vi "Example.vi"() -> ()   [LabVIEW 2019]
uses:
  Test Bench Tools.lvlib
panel:
  in  "Stop":bool
  in  "Launch Test":bool
  out "SerialNumber":string
  out "Test Result":bool
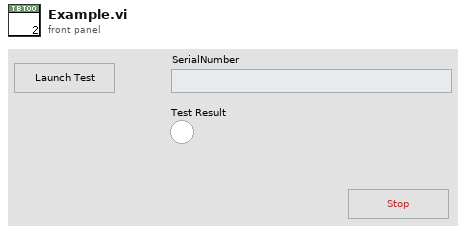
[diagram p1: front panel]
types:
  T1 = enum16{"Station 1", "Station 2", "Station 3", "Station 4"}
  T2 = cluster{"new reference":refnum<k24>, "Array":refnum<k27>[], "Mgessage":refnum<user-event>}
  T3 = enum32{"Invalid", "Standard", "Closed", "Hidden", "Minimized", "Maximized"}
  T4 = enum32{"invalid app kind", "Development System", "Run Time System", "Student Edition", "Embedded LabVIEW", "Evaluation", "Custom"}
  T5 = cluster{"Core":cluster{"Current VI Reference":refnum<vi>, "Close Panel on Exit?":bool}, "Your Boolean data":bool, "Your string data":string, "hWnd":u32}
  T6 = cluster{"Current VI Reference":refnum<vi>, "Close Panel on Exit?":bool}
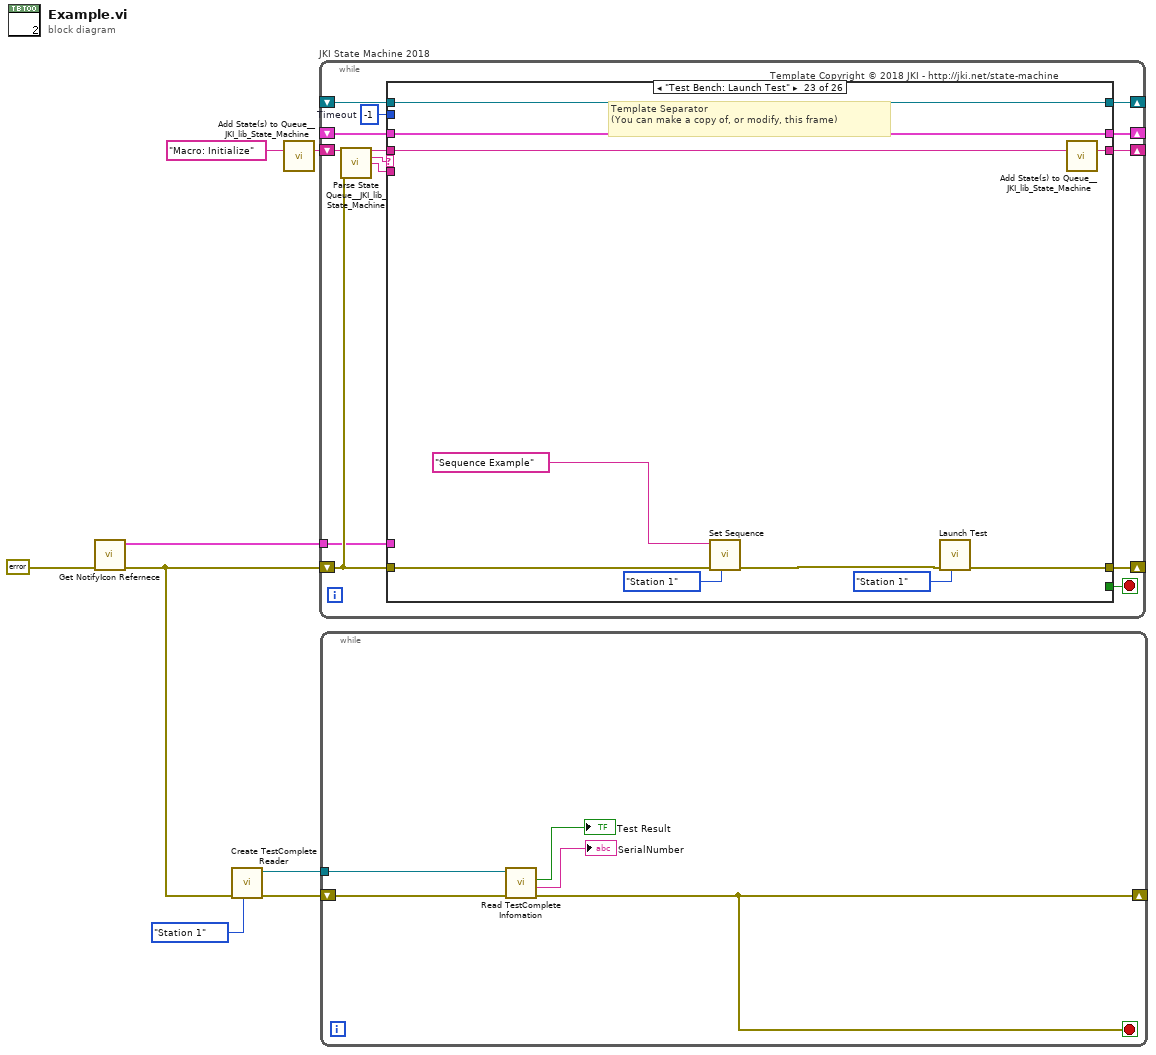
[diagram p0: block diagram]
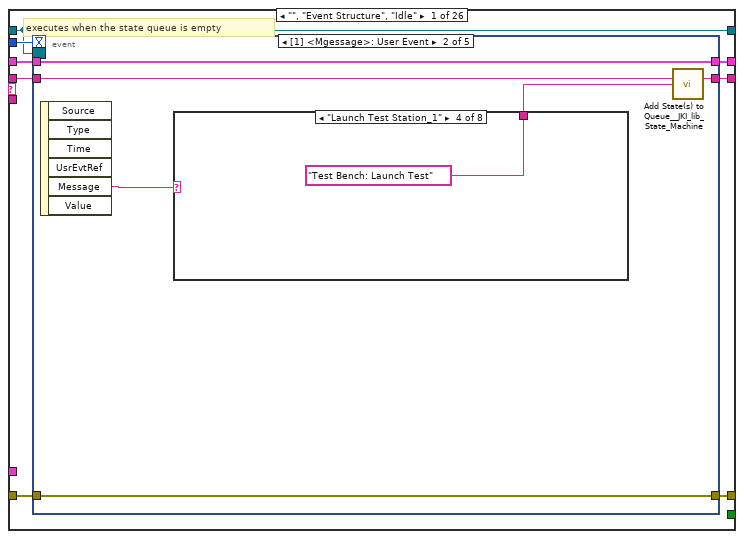
[diagram p2: hidden frame]
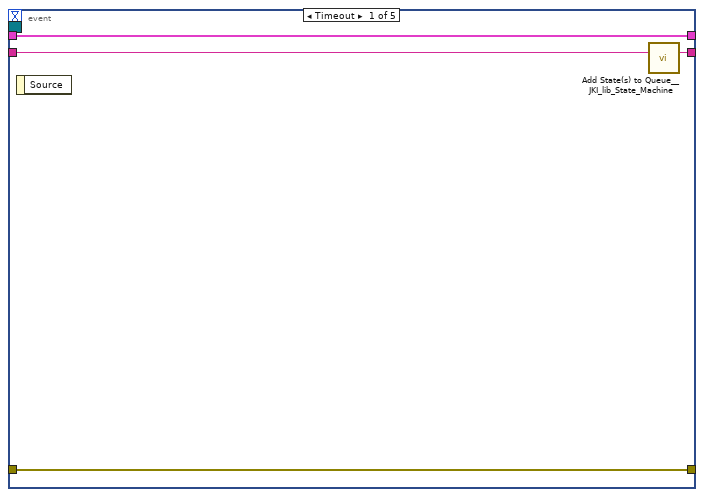
[diagram p3: hidden frame]
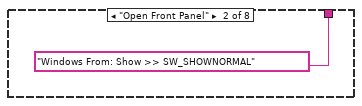
[diagram p5: hidden frame]
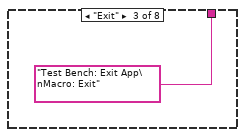
[diagram p6: hidden frame]
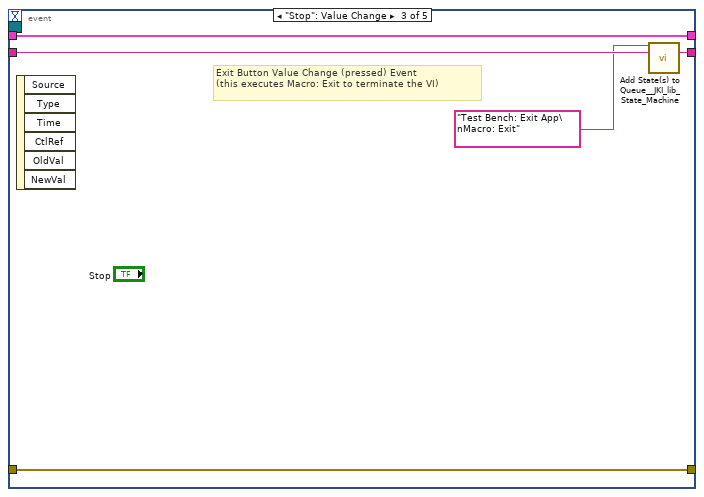
[diagram p11: hidden frame]
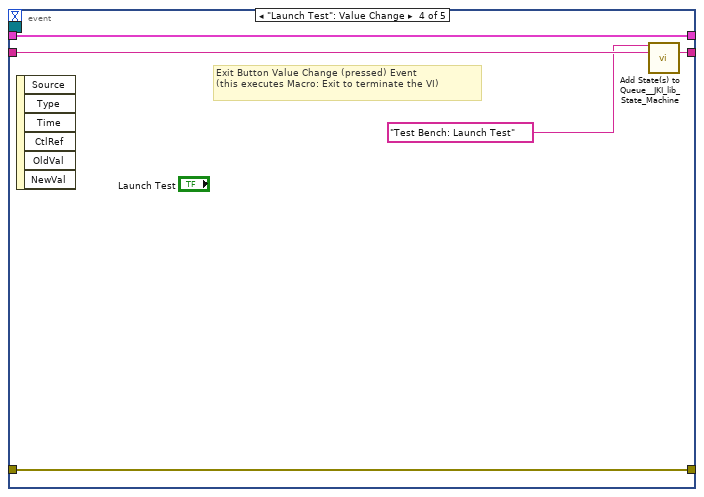
[diagram p12: hidden frame]
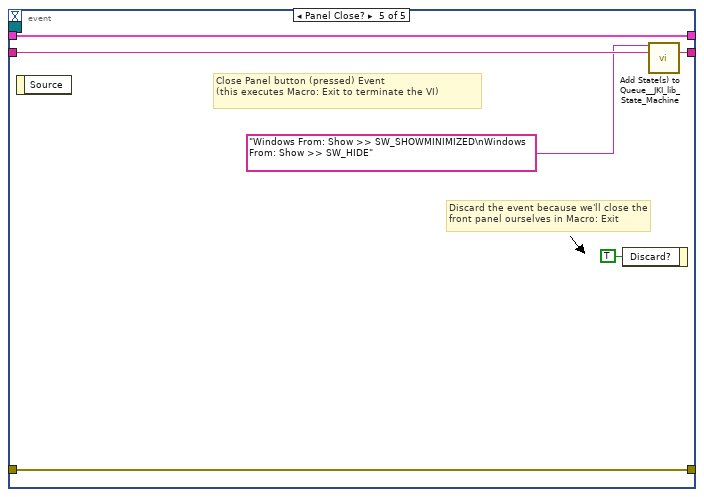
[diagram p13: hidden frame]
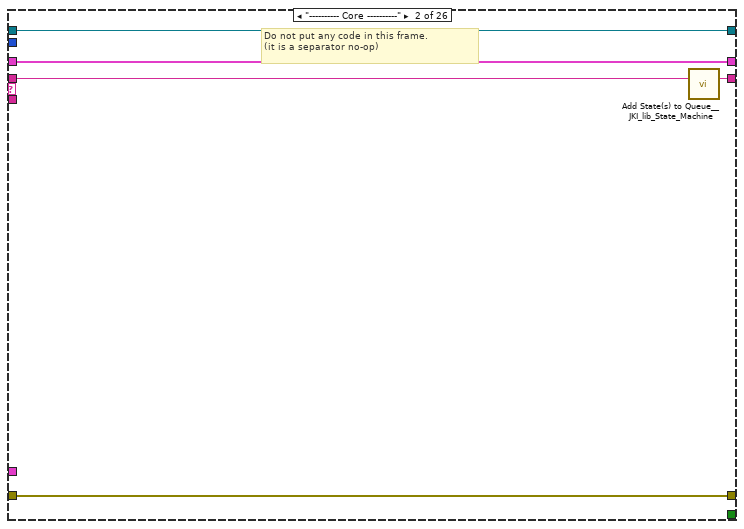
[diagram p14: hidden frame]
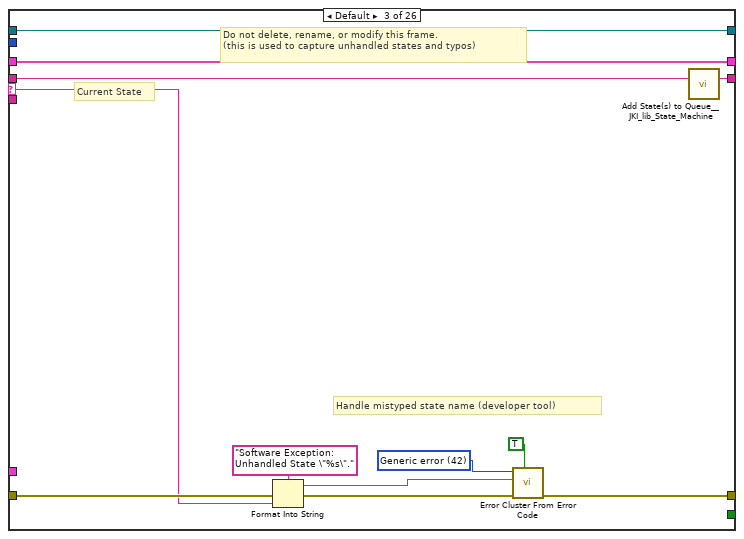
[diagram p15: hidden frame]
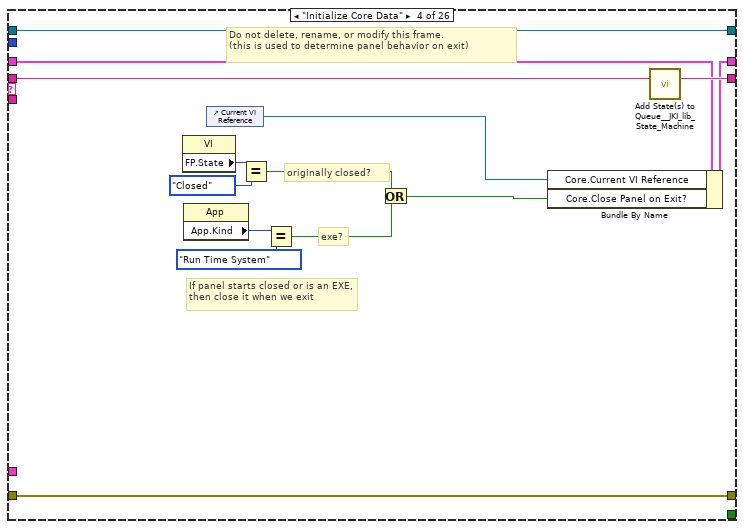
[diagram p16: hidden frame]
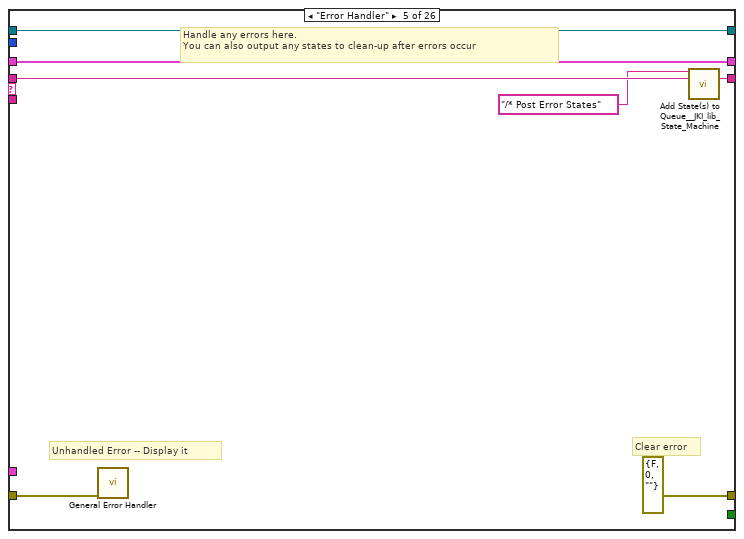
[diagram p17: hidden frame]
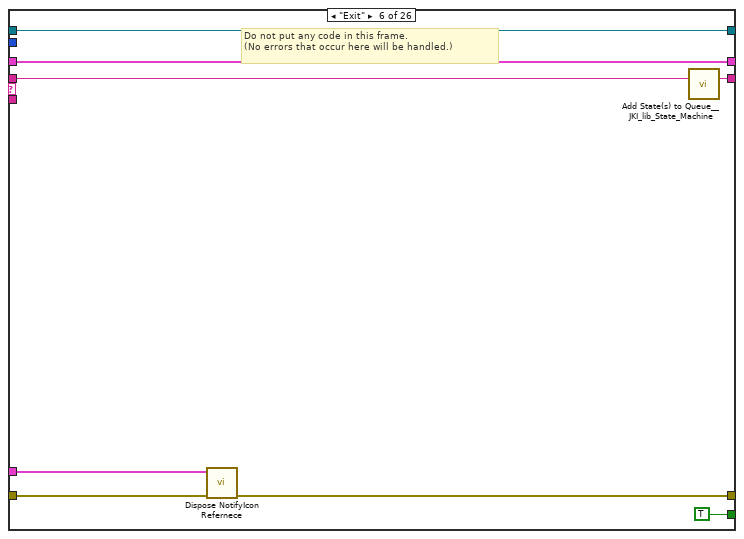
[diagram p18: hidden frame]
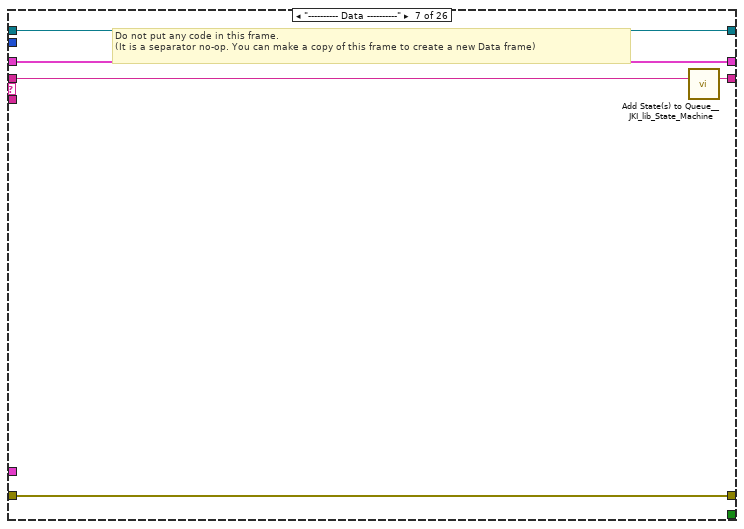
[diagram p19: hidden frame]
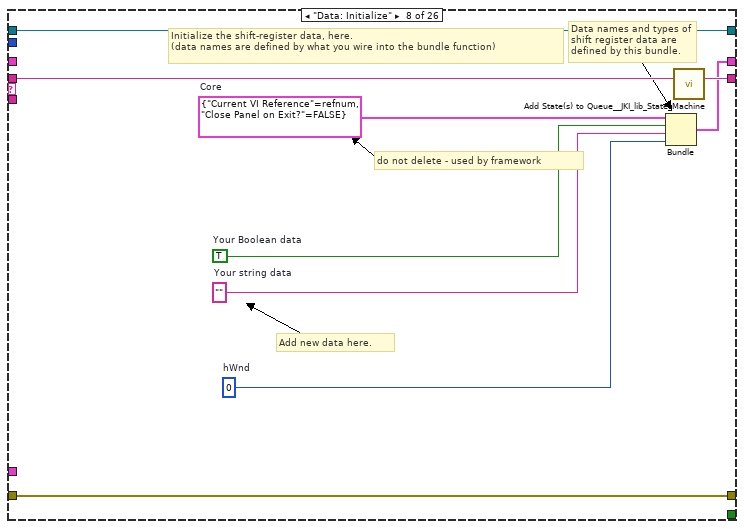
[diagram p20: hidden frame]
diagram:
  n1 = call "Get NotifyIcon Refernece.vi"("error in (no error)"=errorcluster {"status"=FALSE, "code"=0, "source"=""} ("error out")) -> ("error out"=w2:errorcluster, "reference out"=w1:T2)  [unwired: 9 in]
  n2 = call "Create TestComplete Reader.vi"("Station"=T1."Station 1", "error in (no error)"=w2) -> ("error out"=w6:errorcluster, "reader endpoint"=w4:refnum<k21>)  [unwired: 8 in]
  n3 = call <vilib>:"Add State(s) to Queue__JKI_lib_State_Machine.vi"("State(s) in (\"\")"="Macro: Initialize") -> ("States Out"=w8:string)  [unwired: 14 in]
  n4 = while "JKI State Machine 2018" {
    shift-right: [w15] -> _
    shift-left: _ -> [w14]
    shift-right: [w18] -> _
    shift-left: w2 -> [w12]
    shift-right: [w17] -> _
    shift-left: w8 -> [w19]
    shift-right: [w11] -> _
    shift-left: _ -> [w10]
    tunnel: w1 -> [w9]
    stop <- w16 stop-if-true
    w13 = -1  # Timeout
    # "Template Copyright © 2018 JKI - http://jki.net/state-machine"
    n5 = call <vilib>:"Parse State Queue__JKI_lib_State_Machine.vi"("State Queue"=w19, "Error In (no error)"=w12) -> ("Remaining States"=w21:string, "Current State"=w22:string, "Arguments"=w20:string)  [unwired: 11 in]
    n6 = case shown="\"Test Bench: Launch Test\"" w22 {
      selector: w22 -> [_ _ w66 _ _ _ _ _ _ _ _ _ _ _ _ _ _ _ _ _ _ _ _ _ _ _]
      tunnel: w21 -> [w30 w64 w70 w90 w97 w105 w110 w119 w126 w131 w139 w145 w150 w155 w162 w174 w244 w250 w261 w266 w274 w281 w291 w296 w304 w313]
      tunnel: w20 -> [_ _ _ _ _ _ _ _ _ _ _ _ _ _ w157 w168 _ _ _ _ _ _ _ _ w297 _]
      tunnel: w14 -> [w28 w61 w68 w83 w94 w103 w107 _ w121 w128 w137 w143 w147 w153 w160 w170 w241 w247 w258 w263 w272 w279 w289 w293 w299 w307]
      tunnel: [w27 w62 w72 w87 errorcluster {"status"=FALSE, "code"=0, "source"=""} ("error out") w98 w108 w116 w122 w129 w135 w140 w148 w152 w158 w171 w242 w248 w259 w264 w270 w277 w288 w292 w300 w309] -> w18
      tunnel: w12 -> [w26 w62 w71 w87 w93 w99 w108 w116 w123 w129 w134 w141 w148 w152 w159 w172 w242 w248 w259 w264 w271 w278 w285 w292 w301 w310]
      tunnel: [w29 w63 w69 w89 w96 w104 w109 w118 w125 w130 w138 w144 w149 w154 w161 w173 w243 w249 w260 w265 w273 w280 w290 w295 w303 w312] -> w17
      tunnel: [_ _ _ _ _ TRUE _ _ _ _ _ _ _ _ _ _ _ _ _ _ _ _ _ _ _ _] -> w16
      tunnel: [w25 w61 w68 w88 w94 w103 w107 w117 w121 w128 w137 w143 w147 w153 w160 w170 w241 w247 w258 w263 w272 w279 w289 w293 w299 w305] -> w15
      tunnel: w13 -> [w24 _ _ _ _ _ _ _ _ _ _ _ _ _ _ _ _ _ _ _ _ _ _ _ _ _]
      tunnel: [w23 w60 w65 w77 w91 w101 w106 w112 w120 w127 w136 w142 w146 w151 w156 w167 w240 w245 w251 w262 w268 w275 w286 w294 w302 w311] -> w11
      tunnel: w10 -> [w23 w60 w65 w77 w91 w101 w106 w112 w120 w127 _ w142 w146 w151 w156 w167 w240 w245 w251 w262 w268 w275 w286 w294 w302 w311]
      tunnel: w9 -> [_ _ _ _ _ w100 _ _ _ _ w133 _ _ _ _ _ _ _ _ _ _ _ _ _ _ _]
      frame "", "Event Structure", "Idle" {
        # "executes when the state queue is empty"
        n7 = event shown="[1] <Mgessage>: User Event" {
          selector: w23 -> [_ _ _ _ _]
          dyn-events: _ -> [_ _ _ _ _]
          timeout: w24 -> [_ _ _ _ _]
          tunnel: w30 -> [w34 w40 w48 w53 w59]
          tunnel: [w33 w39 w47 w52 w58] -> w29
          tunnel: w28 -> [w31 w37 w45 w50 w56]
          tunnel: [w32 w38 w46 w51 w57] -> w27
          tunnel: w26 -> [w32 w38 w46 w51 w57]
          tunnel: [w31 w37 w45 w50 w56] -> w25
          event Timeout {
            n8 = event-data() -> ()  [unwired: 1 in, 1 out]
            n9 = call <vilib>:"Add State(s) to Queue__JKI_lib_State_Machine.vi"("State(s) in (\"\")"=w34) -> ("States Out"=w33:string)  [unwired: 14 in]
          }
          event User Event {
            n10 = event-data() -> ("Message"=w36:string)  [unwired: 1 in, 5 out]
            n11 = case shown="\"Launch Test Station_1\"" w36 {
              tunnel: [_ "Windows From: Show >> SW_SHOWNORMAL" "Test Bench: Exit App\nMacro: Exit" "Test Bench: Launch Test" _ _ _ _] -> w35
              frame "Idle", Default {
              }
              frame "Open Front Panel" {
              }
              frame "Exit" {
              }
              frame "Launch Test Station_1" {
              }
              frame "Launch Test Station_2" {
              }
              frame "Launch Test Station_3" {
              }
              frame "Launch Test Station_4" {
              }
              frame "Change Product Model" {
              }
            }
            n12 = call <vilib>:"Add State(s) to Queue__JKI_lib_State_Machine.vi"("State(s) in (\"\")"=w40, "State(s) at Back (\"\")"=w35) -> ("States Out"=w39:string)  [unwired: 13 in]
          }
          event "Stop": Value Change {
            # "Exit Button Value Change (pressed) Event\n(this executes Macro: Exit to terminate the VI)"
            n13 = event-data() -> ()  [unwired: 1 in, 6 out]
            n14 = call <vilib>:"Add State(s) to Queue__JKI_lib_State_Machine.vi"("State(s) in Front (\"\")"="Test Bench: Exit App\nMacro: Exit", "State(s) in (\"\")"=w48) -> ("States Out"=w47:string)  [unwired: 13 in]
          }
          event "Launch Test": Value Change {
            # "Exit Button Value Change (pressed) Event\n(this executes Macro: Exit to terminate the VI)"
            n15 = event-data() -> ()  [unwired: 1 in, 6 out]
            n16 = call <vilib>:"Add State(s) to Queue__JKI_lib_State_Machine.vi"("State(s) in Front (\"\")"="Test Bench: Launch Test", "State(s) in (\"\")"=w53) -> ("States Out"=w52:string)  [unwired: 13 in]
          }
          event Panel Close? {
            # "Discard the event because we'll close the front panel ourselves in Macro: Exit"
            # "Close Panel button (pressed) Event\n(this executes Macro: Exit to terminate the VI)"
            n17 = event-data() -> ()  [unwired: 1 in, 1 out]
            n18 = event-data("Discard?"=TRUE) -> ()  [unwired: 1 in, 1 out]
            n19 = call <vilib>:"Add State(s) to Queue__JKI_lib_State_Machine.vi"("State(s) in Front (\"\")"="Windows From: Show >> SW_SHOWMINIMIZED\nWindows From: Show >> SW_HIDE", "State(s) in (\"\")"=w59) -> ("States Out"=w58:string)  [unwired: 13 in]
          }
        }
      }
      frame "---------- Core ----------" {
        # "Do not put any code in this frame.\n(it is a separator no-op)"
        n20 = call <vilib>:"Add State(s) to Queue__JKI_lib_State_Machine.vi"("State(s) in (\"\")"=w64) -> ("States Out"=w63:string)  [unwired: 14 in]
      }
      frame Default {
        w75 = 42 items=["No error", "Argument error", "Memory is full", "Out of zone", "End of file", "File already open", "Generic file I/O error", "File not found", "File permission error", "Disk is full", "Duplicate path", "Too many files open", "System feature not enabled", "Resource file not found", "Cannot add resource", "Resource not found", "Image not found", "Image memory error", "Pen does not exist", "Config type invalid", "Config token not found", "Config parse error", "Config memory error", "Bad external code format", "Bad external code offset", "External code not present", "Null window", "Destroy window error", "Null menu", "Print aborted", "Bad print record", "Print driver error", "Windows error during printing", "Memory error during printing", "Print dialog error", "Generic print error", "Invalid device refnum", "Device not found", "Device parameter error", "Device unit error", "Cannot open device", "Device call aborted", "Generic error", "Cancelled by user", "Object ID too low", "Object ID too high", "Object not in heap", "Unknown heap", "Unknown object (invalid DefProc)", "Unknown object (DefProc not in table)", "Message out of range", "Invalid (null) method", "Unknown message", "Manager call not supported", "Bad address", "Network operation in progress", "Network operation timed out", "Connection is busy", "Network attribute not supported", "Network error", "Address in use", "System out of memory", "Connection aborted", "Connection refused", "Not connected", "Already connected", "Connection closed", "Initialization error (interapplication manager)", "Bad occurrence", "Wait on unbound occurrence handler", "Occurrence queue overflow", "Datalog type conflict", "Unused", "Unrecognized type (interapplication manager)", "Memory corrupt", "Failed to make temporary DLL", "Old CIN version", "Drag socket not found", "Failed to load drop-object", "Failed to register OLE object", "Failed to release OLE object", "Format specifier type mismatch", "Unknown format specifier", "Too few format specifiers", "Too many format specifiers", "Scan failed", "Newer CIN version", "Error converting to variant", "Runtime menu error", "Password tampered", "Variant attribute not found", "Incompatible variant data type", "Event data is not available", "Event Store is not present", "Occurrence is not found", "Event Queue is not created", "Event info is not available", "Refnum passed is NULL", "Error retrieving Class GUID", "Error retrieving CoClass GUID", "Error retrieving TypeLib GUID.", "Bad built application magic bytes.", "Specific driver is different from the specific driver associated with the Logical Name.", "There is no session opened to the class driver.", "Max Error", "MAX - Error with config objects", "MAX - Error loading configuration", "MAX - Group not supported"]
        # "Current State"
        # "Do not delete, rename, or modify this frame.\n(this is used to capture unhandled states and typos)"
        # "Handle mistyped state name (developer tool)"
        n21 = Format Into String(format string="Software Exception: Unhandled State \"%s\"." ("message"), error in=w71, w66) -> (resulting string=w74:string, error out=w73:errorcluster)  [unwired: 1 in]
        n22 = call <vilib>:"Error Cluster From Error Code.vi"("show call chain? (False)"=TRUE, "error in (no error)"=w73, "error message (\"\")"=w74, "error code (0)"=w75) -> ("error out"=w72:errorcluster)  [unwired: 5 in]
        n23 = call <vilib>:"Add State(s) to Queue__JKI_lib_State_Machine.vi"("State(s) in (\"\")"=w70) -> ("States Out"=w69:string)  [unwired: 14 in]
      }
      frame "Initialize Core Data" {
        # "Do not delete, rename, or modify this frame.\n(this is used to determine panel behavior on exit)"
        # "originally closed?"
        # "exe?"
        # "If panel starts closed or is an EXE, then close it when we exit"
        n24 = property class="VI"() -> ("FP.State"=w80:T3)  [unwired: 2 in, 2 out]
        n25 = property class="App"() -> ("App.Kind"=w86:T4)  [unwired: 2 in, 2 out]
        n26 = control-ref of="Current VI Reference"() -> (w81:refnum<vi>)
        n27 = Equal?(x=w80, y=T3."Closed" ("Front Panel Window:State")) -> (x = y?=w78:bool)
        n28 = Equal?(x=w86, y=T4."Run Time System" ("Application:Kind")) -> (x = y?=w84:bool)
        n29 = Or(x=w78, y=w84) -> (x .or. y?=w82:bool)
        n30 = Bundle By Name(cluster=w83, "Core.Current VI Reference"=w81, "Core.Close Panel on Exit?"=w82) -> (w88:T5)
        n31 = call <vilib>:"Add State(s) to Queue__JKI_lib_State_Machine.vi"("State(s) in (\"\")"=w90) -> ("States Out"=w89:string)  [unwired: 14 in]
      }
      frame "Error Handler" {
        # "Unhandled Error -- Display it"
        # "Handle any errors here.\nYou can also output any states to clean-up after errors occur"
        # "Clear error"
        n32 = call <vilib>:"General Error Handler.vi"("error in (no error)"=w93) -> ()  [unwired: 10 in, 5 out]
        n33 = call <vilib>:"Add State(s) to Queue__JKI_lib_State_Machine.vi"("State(s) in Front (\"\")"="/* Post Error States", "State(s) in (\"\")"=w97) -> ("States Out"=w96:string)  [unwired: 13 in]
      }
      frame "Exit" {
        # "Do not put any code in this frame.\n(No errors that occur here will be handled.)"
        n34 = call "Dispose NotifyIcon Refernece.vi"("error in (no error)"=w99, "reference"=w100) -> ("error out"=w98:errorcluster)  [unwired: 9 in]
        n35 = call <vilib>:"Add State(s) to Queue__JKI_lib_State_Machine.vi"("State(s) in (\"\")"=w105) -> ("States Out"=w104:string)  [unwired: 14 in]
      }
      frame "---------- Data ----------" {
        # "Do not put any code in this frame.\n(It is a separator no-op. You can make a copy of this frame to create a new Data frame)"
        n36 = call <vilib>:"Add State(s) to Queue__JKI_lib_State_Machine.vi"("State(s) in (\"\")"=w110) -> ("States Out"=w109:string)  [unwired: 14 in]
      }
      frame "Data: Initialize" {
        w111 = u32 0  # hWnd
        w113 = T6 {"Current VI Reference"=refnum, "Close Panel on Exit?"=FALSE}  # Core
        w115 = TRUE  # Your Boolean data
        w114 = ""  # Your string data
        # "do not delete - used by framework"
        # "Add new data here."
        # "Data names and types of shift register data are defined by this bundle."
        # "Initialize the shift-register data, here.\n(data names are defined by what you wire into the bundle function)"
        n37 = Bundle("Core"=w113, "Your Boolean data"=w115, "Your string data"=w114, "hWnd"=w111) -> (w117:T5)  [unwired: 1 in]
        n38 = call <vilib>:"Add State(s) to Queue__JKI_lib_State_Machine.vi"("State(s) in (\"\")"=w119) -> ("States Out"=w118:string)  [unwired: 14 in]
      }
      frame "Data: Cleanup" {
        # "Cleanup any data and references, here.\n(this is called automatically, by the Macro: Exit)"
        n39 = Unbundle By Name(w121) -> ("Core.Current VI Reference"=w124:refnum<vi>)
        n40 = Close Reference(reference=w124, error in (no error)=w123) -> (error out=w122:errorcluster)
        n41 = call <vilib>:"Add State(s) to Queue__JKI_lib_State_Machine.vi"("State(s) in (\"\")"=w126) -> ("States Out"=w125:string)  [unwired: 14 in]
      }
      frame "---------- Events ----------" {
        # "Do not put any code in this frame.\n(It is a separator no-op. You can make a copy of this frame to create a new UI frame)"
        n42 = call <vilib>:"Add State(s) to Queue__JKI_lib_State_Machine.vi"("State(s) in (\"\")"=w131) -> ("States Out"=w130:string)  [unwired: 14 in]
      }
      frame "Events: Register" {
        # "Do not put any code in this frame.\n(It is a separator no-op. You can make a copy of this frame to create a new UI frame)"
        n43 = Unbundle By Name(w133) -> ("Mgessage"=w132:refnum<user-event>)
        n44 = register-events(error in=w134, w132) -> (reference out=w136:refnum<event-registration>, error out=w135:errorcluster)  [unwired: 1 in]
        n45 = call <vilib>:"Add State(s) to Queue__JKI_lib_State_Machine.vi"("State(s) in (\"\")"=w139) -> ("States Out"=w138:string)  [unwired: 14 in]
      }
      frame "Events: Unregister" {
        # "Do not put any code in this frame.\n(It is a separator no-op. You can make a copy of this frame to create a new UI frame)"
        n46 = Unregister For Events(event registration refnum=w142, error in=w141) -> (error out=w140:errorcluster)
        n47 = call <vilib>:"Add State(s) to Queue__JKI_lib_State_Machine.vi"("State(s) in (\"\")"=w145) -> ("States Out"=w144:string)  [unwired: 14 in]
      }
      frame "---------- UI ----------" {
        # "Do not put any code in this frame.\n(It is a separator no-op. You can make a copy of this frame to create a new UI frame)"
        n48 = call <vilib>:"Add State(s) to Queue__JKI_lib_State_Machine.vi"("State(s) in (\"\")"=w150) -> ("States Out"=w149:string)  [unwired: 14 in]
      }
      frame "UI: Initialize" {
        # "Initialize the User Interface, here.\n(this is called automatically, by the Macro: Init)"
        n49 = call <vilib>:"Add State(s) to Queue__JKI_lib_State_Machine.vi"("State(s) in (\"\")"=w155) -> ("States Out"=w154:string)  [unwired: 14 in]
      }
      frame "UI: Cursor Set" {
        # "Argument"
        # "Set and Unset Cursor Busy.\n(Usage: \"UI: Cursor Set >> Busy|Idle\")"
        n50 = case shown="\"Idle\", Default" w157 {
          tunnel: w159 -> [w164 w166]
          tunnel: [w163 w165] -> w158
          frame "Idle", Default {
            n51 = call <vilib>:"Unset Busy.vi"("error in (no error)"=w164) -> ("error out"=w163:errorcluster)  [unwired: 10 in]
          }
          frame "Busy" {
            n52 = call <vilib>:"Set Busy.vi"("error in (no error)"=w166) -> ("error out"=w165:errorcluster)  [unwired: 9 in, 1 out]
          }
        }
        n53 = call <vilib>:"Add State(s) to Queue__JKI_lib_State_Machine.vi"("State(s) in (\"\")"=w162) -> ("States Out"=w161:string)  [unwired: 14 in]
      }
      frame "UI: Front Panel State" {
        # "Argument"
        # "Set Front Panel Open or Closed\n(Usage: \"UI: Front Panel State >> Open|Close\")"
        n54 = Unbundle By Name(w170) -> ("Core.Current VI Reference"=w169:refnum<vi>)
        n55 = case shown="\"Minimize\", \"Minimized\"" w168 {
          tunnel: w172 -> [w180 w195 w206 w219 w232]
          tunnel: [w182 w196 w208 w221 w234] -> w171
          tunnel: w169 -> [w181 w193 w207 w220 w233]
          frame "Open", "Standard", Default {
            w175 = T3."Standard" ("State")
            n56 = property class="VI"(reference=w181, error in=w180) -> (reference out=w178:refnum<vi>, error out=w179:errorcluster, "FP.State"=w177:T3)
            n57 = Not Equal?(x=w177, y=w175) -> (x != y?=w176:bool)
            n58 = case shown="True" w176 {
              tunnel: [w186 w188] -> w182
              tunnel: w179 -> [w185 w188]
              tunnel: w178 -> [w184 _]
              tunnel: w175 -> [w183 _]
              frame True {
                n59 = invoke class="VI" method="FP.Open"(reference=w184, error in=w185, "Activate"=TRUE, "State"=w183) -> (error out=w186:errorcluster)  [unwired: 1 in, 4 out]
              }
              frame False {
              }
            }
          }
          frame "Close", "Closed" {
            n60 = property class="VI"(reference=w193, error in=w195) -> (reference out=w192:refnum<vi>, error out=w194:errorcluster, "FP.State"=w190:T3)
            n61 = Not Equal?(x=w190, y=T3."Closed" ("Front Panel Window:State")) -> (x != y?=w189:bool)
            n62 = case shown="True" w189 {
              tunnel: [w197 w200] -> w196
              tunnel: w194 -> [w197 w199]
              tunnel: w192 -> [_ w198]
              frame False {
              }
              frame True {
                n63 = invoke class="VI" method="FP.Close"(reference=w198, error in=w199) -> (error out=w200:errorcluster)  [unwired: 1 in, 2 out]
              }
            }
          }
          frame "Hidden", "Hide" {
            w201 = T3."Hidden" ("State")
            n64 = property class="VI"(reference=w207, error in=w206) -> (reference out=w204:refnum<vi>, error out=w205:errorcluster, "FP.State"=w203:T3)
            n65 = Not Equal?(x=w203, y=w201) -> (x != y?=w202:bool)
            n66 = case shown="True" w202 {
              tunnel: [w212 w213] -> w208
              tunnel: w205 -> [w211 w213]
              tunnel: w204 -> [w210 _]
              tunnel: w201 -> [w209 _]
              frame True {
                n67 = invoke class="VI" method="FP.Open"(reference=w210, error in=w211, "State"=w209) -> (error out=w212:errorcluster)  [unwired: 2 in, 4 out]
              }
              frame False {
              }
            }
          }
          frame "Minimize", "Minimized" {
            w214 = T3."Minimized" ("State")
            n68 = property class="VI"(reference=w220, error in=w219) -> (reference out=w217:refnum<vi>, error out=w218:errorcluster, "FP.State"=w216:T3)
            n69 = Not Equal?(x=w216, y=w214) -> (x != y?=w215:bool)
            n70 = case shown="True" w215 {
              tunnel: [w225 w226] -> w221
              tunnel: w218 -> [w224 w226]
              tunnel: w217 -> [w223 _]
              tunnel: w214 -> [w222 _]
              frame True {
                n71 = invoke class="VI" method="FP.Open"(reference=w223, error in=w224, "State"=w222) -> (error out=w225:errorcluster)  [unwired: 2 in, 4 out]
              }
              frame False {
              }
            }
          }
          frame "Maximize", "Maximized" {
            w227 = T3."Maximized" ("State")
            n72 = property class="VI"(reference=w233, error in=w232) -> (reference out=w230:refnum<vi>, error out=w231:errorcluster, "FP.State"=w229:T3)
            n73 = Not Equal?(x=w229, y=w227) -> (x != y?=w228:bool)
            n74 = case shown="True" w228 {
              tunnel: [w238 w239] -> w234
              tunnel: w231 -> [w237 w239]
              tunnel: w230 -> [w236 _]
              tunnel: w227 -> [w235 _]
              frame True {
                n75 = invoke class="VI" method="FP.Open"(reference=w236, error in=w237, "State"=w235) -> (error out=w238:errorcluster)  [unwired: 2 in, 4 out]
              }
              frame False {
              }
            }
          }
        }
        n76 = call <vilib>:"Add State(s) to Queue__JKI_lib_State_Machine.vi"("State(s) in (\"\")"=w174) -> ("States Out"=w173:string)  [unwired: 14 in]
      }
      frame "---------- Macro ----------" {
        # "Do not put any code in this frame.\n(It is a separator no-op. You can make a copy of this frame to create a new Macro frame)"
        n77 = call <vilib>:"Add State(s) to Queue__JKI_lib_State_Machine.vi"("State(s) in (\"\")"=w244) -> ("States Out"=w243:string)  [unwired: 14 in]
      }
      frame "Macro: Initialize" {
        # "Initialization Macro\n(This is called once, when the VI starts)"
        n78 = call <vilib>:"Add State(s) to Queue__JKI_lib_State_Machine.vi"("State(s) in Front (\"\")"="Data: Initialize\nInitialize Core Data\nEvents: Register\nUI: Initialize\nUI: Front Panel State >> Open\nTest Bench: Launch Test Bench\nWindows From: Find Windows\nWindows From: Show >> SW_SHOWMINIMIZED\nWindows From: Show >> SW_HIDE", "State(s) in (\"\")"=w250) -> ("States Out"=w249:string)  [unwired: 13 in]
      }
      frame "Macro: Exit" {
        # "Exit Macro\n(This is called once, when the VI exits)"
        n79 = Unbundle By Name(w258) -> ("Core.Close Panel on Exit?"=w257:bool)
        n80 = Select(t="UI: Front Panel State >> Close", s=w257, f="") -> (s? t:f=w254:string)
        n81 = call <vilib>:"Add State(s) to Queue__JKI_lib_State_Machine.vi"("State(s) in (\"\")"=w254, "State(s) at Back (\"\")"="Data: Cleanup\nEvents: Unregister\nExit") -> ("States Out"=w252:string)  [unwired: 13 in]
        n82 = call <vilib>:"Add State(s) to Queue__JKI_lib_State_Machine.vi"("State(s) in Front (\"\")"=w252, "State(s) in (\"\")"=w261) -> ("States Out"=w260:string)  [unwired: 13 in]
      }
      frame "---------- Test Bench ----------" {
        # "Template Separator\n(You can make a copy of, or modify, this frame)"
        n83 = call <vilib>:"Add State(s) to Queue__JKI_lib_State_Machine.vi"("State(s) in (\"\")"=w266) -> ("States Out"=w265:string)  [unwired: 14 in]
      }
      frame "Test Bench: Launch Test Bench" {
        # "Template Separator\n(You can make a copy of, or modify, this frame)"
        n84 = call "Launch Test Bench.vi"("Station"=T1."Station 1", "error in (no error)"=w271, "App Path"=path "C:/Program Files (x86)/National Instruments/LabVIEW 2019/resource/Framework/Providers/Test Bench/TestBench.exe") -> ("error out"=w270:errorcluster)  [unwired: 8 in]
        n85 = call <vilib>:"Add State(s) to Queue__JKI_lib_State_Machine.vi"("State(s) in (\"\")"=w274) -> ("States Out"=w273:string)  [unwired: 14 in]
      }
      frame "Test Bench: Exit App" {
        # "Template Separator\n(You can make a copy of, or modify, this frame)"
        n86 = call "Exit Test Bench.vi"("Station"=T1."Station 1", "error in (no error)"=w278) -> ("error out"=w277:errorcluster)  [unwired: 9 in]
        n87 = call <vilib>:"Add State(s) to Queue__JKI_lib_State_Machine.vi"("State(s) in (\"\")"=w281) -> ("States Out"=w280:string)  [unwired: 14 in]
      }
      frame "Test Bench: Launch Test" {
        # "Template Separator\n(You can make a copy of, or modify, this frame)"
        n88 = call "Set Sequence.vi"("Station"=T1."Station 1", "error in (no error)"=w285, "Sequence"="Sequence Example" ("Info")) -> ("error out"=w284:errorcluster)  [unwired: 8 in]
        n89 = call "Launch Test.vi"("Station"=T1."Station 1", "error in (no error)"=w284) -> ("error out"=w288:errorcluster)  [unwired: 9 in]
        n90 = call <vilib>:"Add State(s) to Queue__JKI_lib_State_Machine.vi"("State(s) in (\"\")"=w291) -> ("States Out"=w290:string)  [unwired: 14 in]
      }
      frame "---------- Windows From ----------" {
        # "Template Separator\n(You can make a copy of, or modify, this frame)"
        n91 = call <vilib>:"Add State(s) to Queue__JKI_lib_State_Machine.vi"("State(s) in (\"\")"=w296) -> ("States Out"=w295:string)  [unwired: 14 in]
      }
      frame "Windows From: Show" {
        # "Template Separator\n(You can make a copy of, or modify, this frame)"
        n92 = Unbundle By Name(w299) -> ("hWnd"=w298:u32)
        n93 = call "Show Windows.vi"("nCmdShow"=w297, "error in (no error)"=w301, "hWnd"=w298) -> ("error out"=w300:errorcluster)  [unwired: 7 in, 1 out]
        n94 = call <vilib>:"Add State(s) to Queue__JKI_lib_State_Machine.vi"("State(s) in (\"\")"=w304) -> ("States Out"=w303:string)  [unwired: 14 in]
      }
      frame "Windows From: Find Windows" {
        # "Template Separator\n(You can make a copy of, or modify, this frame)"
        n95 = Unbundle By Name(w307) -> ("Core.Current VI Reference"=w308:refnum<vi>)
        n96 = call "Find Windows.vi"("error in (no error)"=w310, "VI reference"=w308) -> ("error out"=w309:errorcluster, "hWnd"=w306:u32)  [unwired: 8 in]
        n97 = Bundle By Name(cluster=w307, "hWnd"=w306) -> (w305:T5)
        n98 = call <vilib>:"Add State(s) to Queue__JKI_lib_State_Machine.vi"("State(s) in (\"\")"=w313) -> ("States Out"=w312:string)  [unwired: 14 in]
      }
    }
  }
  n99 = while {
    tunnel: w4 -> [w318]
    shift-right: [w316] -> _
    shift-left: w6 -> [w317]
    stop <- w316 stop-if-true
    n100 = call "Read TestComplete Infomation.vi"("error in (no error)"=w317, "endpoint in"=w318) -> ("error out"=w316:errorcluster, "SerialNumber"=→"SerialNumber":string, "Test Result"=→"Test Result":bool)  [unwired: 5 in, 2 out]
  }
